vi "日志信息主动发送(子VI).vi"   [LabVIEW 2016, in "数据传输系统-03.lvlib"]
types:
  T1 = typedef "LVDateTimeRec.ctl" = cluster{"秒数的小数部分":dbl, "秒":i32, "分":i32, "时":i32, "日":i32, "月":i32, "年":i32, "天数（周）":i32, "天数（年）":i32, "DST":i32}
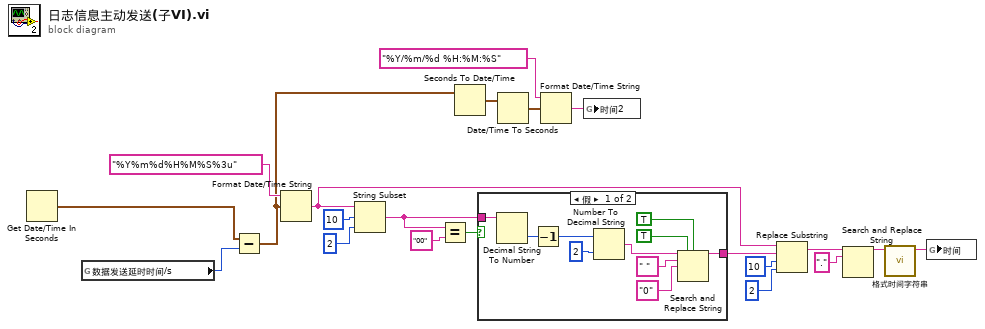
[diagram p0: block diagram]
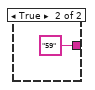
[diagram p2: hidden frame]
diagram:
  n1 = Get Date/Time In Seconds() -> (seconds since 1Jan1904=w2:timestamp)
  n2 = global read "断电保存全局.vi" "数据发送延时时间/s"() -> (w3:i32)
  n3 = Subtract(x=w2, y=w3) -> (x-y=w1:timestamp)
  n4 = Format Date/Time String(time format string (%c)="%Y%m%d%H%M%S%3u" ("时间格式字符串(%c)"), seconds (now)=w1) -> (date/time string=w10:string)  [unwired: 1 in]
  n5 = String Subset(string=w10, offset (0)=10 ("偏移量(0)"), length (rest)=2 ("长度（子字符串长度）")) -> (substring=w18:string)
  n6 = Equal?(x=w18, y="00") -> (x = y?=w17:bool)
  n7 = Seconds To Date/Time(time stamp (now)=w1) -> (date time rec=w7:T1)  [unwired: 1 in]
  n8 = case shown="假" w17 {
    tunnel: w18 -> [w31 _]
    tunnel: [w23 "59" ("y")] -> w19
    frame False {
      n9 = Decimal String To Number(string=w31) -> (number=w30:i32)  [unwired: 2 in, 1 out]
      n10 = Decrement(x=w30) -> (x-1=w24:i32)
      n11 = Number To Decimal String(number=w24, width (-)=i16 2 ("宽度(-)")) -> (decimal integer string=w26:string)
      n12 = Search and Replace String(replace all?=TRUE ("替换全部？(F)"), case sensitive?=TRUE ("忽略大小写？(F)"), input string=w26, search string=" " ("搜索字符串"), replace string="0" ("替换字符串(\"\")")) -> (result string=w23:string)  [unwired: 3 in, 3 out]
    }
    frame True {
    }
  }
  n13 = Date/Time To Seconds(2:w7) -> (0:w9:timestamp)  [unwired: 1 in]
  n14 = Format Date/Time String(time format string (%c)="%Y/%m/%d %H:%M:%S" ("时间格式字符串(%c)"), seconds (now)=w9) -> (date/time string=w6:string)  [unwired: 1 in]
  n15 = global write "全局 时间2.vi" "时间2"(w6) -> ()
  n16 = Replace Substring(2:2 ("长度（子字符串长度）"), 3:10 ("偏移量(0)"), 4:w19, 5:w10) -> (1:w11:string)  [unwired: 1 out]
  n17 = Search and Replace String(input string=w11, search string="." ("搜索字符串")) -> (result string=w4:string)  [unwired: 6 in, 3 out]
  n18 = call "格式时间字符串.vi"("字符串"=w4) -> ("连接的字符串"=w12:string)  [unwired: 10 in]
  n19 = global write "全局 水样时间.vi" "时间"(w12) -> ()
